vi "Check Is Test Case.vi"(11 "reference in":refnum<vi>) -> (2 "Is Test Case?":bool, 3 "reference out":refnum<vi>)   [LabVIEW 2020, in "Icon Decorator.lvlib" / "Icon Decorator.lvclass"]
uses:
  Icon Decorator.lvclass
  LUnit Test Case.lvclass
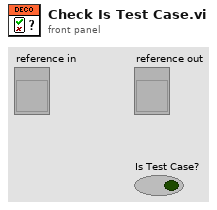
[diagram p1: front panel]
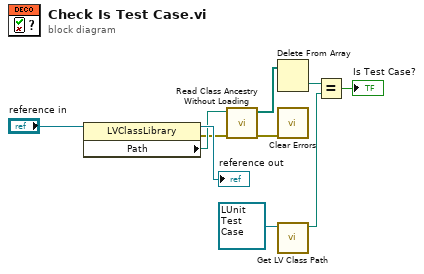
[diagram p0: block diagram]
diagram:
  n1 = property class="LVClassLibrary"(reference="reference in") -> (reference out=→"reference out":refnum<vi>, error out=w6:errorcluster, "Path"=w7:path)  [unwired: 1 in]
  n2 = call <vilib>:"Read Class Ancestry Without Loading.vi"("error in (no error)"=w6, "LabVIEW Class Path"=w7) -> ("error out"=w5:errorcluster, "Class Ancestry"=w4:path[])  [unwired: 8 in]
  n3 = Delete From Array(array=w4) -> (deleted portion=w3:path)  [unwired: 2 in, 1 out]
  n4 = call <vilib>:"Clear Errors.vi"("error in (no error)"=w5) -> ()  [unwired: 5 in, 2 out]
  n5 = call <vilib>:"Get LV Class Path.vi"("object"=refnum<class "LUnit Test Case.lvclass"> refnum ("LUnit Test Case V2.lvclass")) -> ("class path"=w2:path)  [unwired: 9 in, 1 out]
  n6 = Equal?(x=w3, y=w2) -> (x = y?=→"Is Test Case?":bool)
